vi "oa_Get the Index of the 1st Point in One Cycle (N Channels).vi"(0 "resampled signal":cluster{"r0":dbl, "dr":dbl, "Y":dbl[]}[](array[cluster]) {"r0" format="%.2p"; "dr" format="%.2p"; "Y" format="%.2f"}, 1 "reset? (True)":bool=TRUE, 7 "speed profile":T1 {"speed [RPM]" format="%.2f"; "time [s]" format="%.2f"}, 9 "interpolated pulse positions":dbl[](array[numeric]) format="%.2f", 11 "error in (no error)":errorcluster, 12 "index mode":u16(ring) items=["round to nearest", "round to ceiling"]) -> (4 "resampled signal out":cluster{"r0":dbl, "dr":dbl, "Y":dbl[]}[](array[cluster]) {"r0" format="%.2p"; "dr" format="%.2p"; "Y" format="%.2f"}, 10 "interpolated pulse positions out":dbl[](array[numeric]), 15 "error out":errorcluster)   [LabVIEW 2017, in "SoundVib_Resampling.lvlib"]
uses:
  <vilib>/addons/Sound and Vibration/Order Analysis/Resample Order Tracking/SoundVib_Resampling.lvlib
  <vilib>/addons/Sound and Vibration/Order Analysis/Tach Process/SubVIs/speed profile.ctl
  <vilib>/addons/Sound and Vibration/Order Analysis/Tach Process/SoundVib_TachProcess.lvlib
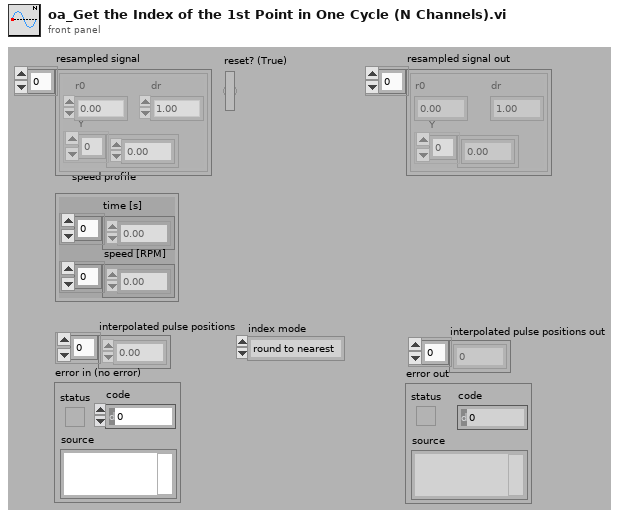
[diagram p1: front panel]
types:
  T1 = typedef "SoundVib_TachProcess.lvlib/speed profile.ctl" = cluster{"time [s]":dbl[], "speed [RPM]":dbl[]}
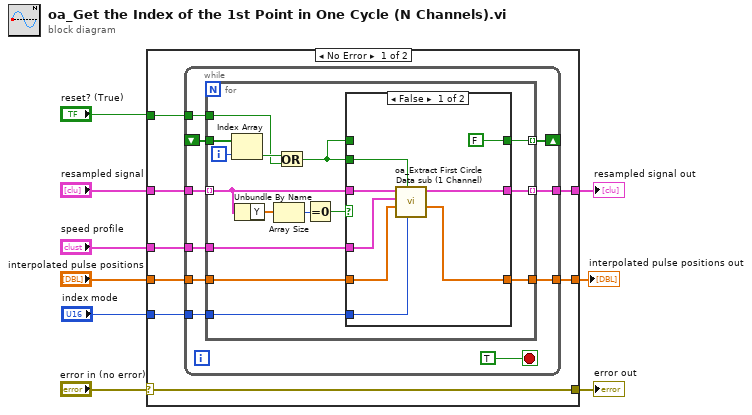
[diagram p0: block diagram]
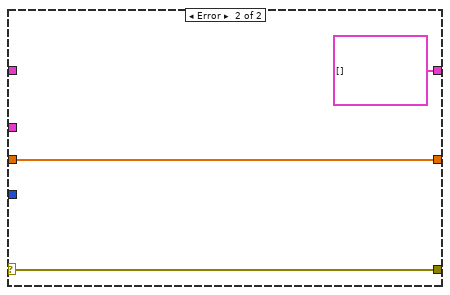
[diagram p3: hidden frame]
diagram:
  n1 = case shown="No Error" "error in (no error)" {
    selector: "error in (no error)" -> [w12 w56]
    tunnel: [w12 w56] -> w6
    tunnel: "reset? (True)" -> [w17 _]
    tunnel: "resampled signal" -> [w16 _]
    tunnel: [w15 cluster{"r0":dbl, "dr":dbl, "Y":dbl[]}[] []] -> w4
    tunnel: "speed profile" -> [w14 _]
    tunnel: "interpolated pulse positions" -> [w13 w54]
    tunnel: [w11 w54] -> w2
    tunnel: "index mode" -> [w10 _]
    frame No Error {
      n2 = while {
        tunnel: w17 -> [w27]
        tunnel: w16 -> [w26]
        tunnel: [w25] -> w15
        tunnel: w14 -> [w24]
        tunnel: w13 -> [w23]
        shift-right: [w22] -> _
        shift-left: _ -> [w21]
        tunnel: [w19] -> w11
        tunnel: w10 -> [w18]
        stop <- TRUE stop-if-true
        n3 = for {
          tunnel: w27 -> [w31]
          tunnel: w26 -> [w39] mode=indexing
          tunnel: [w40] -> w25 mode=indexing
          tunnel: w24 -> [w42]
          tunnel: w23 -> [w41]
          tunnel: [w35] -> w22 mode=indexing
          tunnel: w21 -> [w34]
          tunnel: [w29] -> w19
          tunnel: w18 -> [w28]
          i -> [w33]
          n4 = Index Array(array=w34, index=w33) -> (element=w32:bool)
          n5 = Unbundle By Name(w39) -> ("Y"=w38:dbl[])
          n6 = Array Size(array=w38) -> (size(s)=w37:i32)
          n7 = Or(x=w32, y=w31) -> (x .or. y?=w30:bool)
          n8 = Equal To 0?(x=w37) -> (x = 0?=w36:bool)
          n9 = case shown="False" w36 {
            tunnel: w42 -> [w50 _]
            tunnel: w41 -> [w49 w51]
            tunnel: [w48 w52] -> w40
            tunnel: w39 -> [w47 w52]
            tunnel: [FALSE w53] -> w35
            tunnel: w30 -> [w45 _]
            tunnel: w30 -> [_ w53]
            tunnel: [w44 w51] -> w29
            tunnel: w28 -> [w43 _]
            frame False {
              n10 = call <vilib>:"oa_Extract First Circle Data sub (1 Channel).vi"("index mode"=w43, "reset? (True)"=w45, "interpolated pulse positions"=w49, "speed profile"=w50, "resampled signal"=w47) -> ("interpolated pulse positions out"=w44:dbl[], "resampled signal out"=w48:cluster{"r0":dbl, "dr":dbl, "Y":dbl[]})  [unwired: 5 in]
            }
            frame True {
            }
          }
        }
      }
    }
    frame Error {
    }
  }
  "error out" <- w6
  "resampled signal out" <- w4
  "interpolated pulse positions out" <- w2
